vi "MiPS_switch_heater.vi"(0 "ref_big_msg":refnum<vi>, 1 "ref_shim_relay_ch1":refnum<vi>, 2 "ref_shim_relay_ch2":refnum<vi>, 4 "ref_shim_relay_status":refnum<vi>, 5 "error in":errorcluster, 6 "ref_timeout_slider":refnum<vi>, 7 "heater_status_now":bool, 8 "ref_in":T1, 9 "ISOBUS address":T4, 10 "switching_allowed":bool, 11 "conn_id_in":refnum<k5>) -> (13 "conn_id_out":refnum<k5>, 14 "ref_out":T1, 19 "error out":errorcluster)   [LabVIEW 2019]
uses:
  Mercury iXX Modules/Public/Controls/ISOBus Address.ctl
  Mercury iXX Modules/Public/Controls/Mercury Reference.ctl
  Mercury iXX Modules/Public/Controls/Comms Transport Layer.ctl
  Mercury iXX Modules/Private/Controls/Query Dynamic Reference.ctl
  Mercury iXX Modules/Public/Libraries/Magnet/Controls/Switch Heater.ctl
  Mercury iXX Modules/Public/Libraries/Magnet/Signals/Set/Switch Heater No Check (Set).vi
  Mercury iXX Modules/Public/Libraries/Magnet.lvlib
  Mercury iXX Modules/Mercury iXX.lvlib
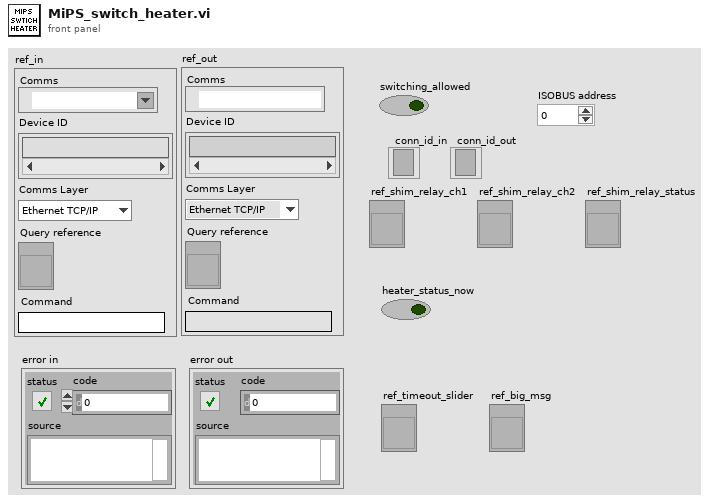
[diagram p1: front panel]
types:
  T1 = typedef "Mercury iXX.lvlib/Mercury Reference.ctl" = cluster{"Comms":refnum<visa-resource-name>, "Device ID":string[], "Comms Layer":T2, "Command":string, "Query reference":T3}
  T2 = typedef "Mercury iXX.lvlib/Comms Transport Layer.ctl" = enum16{"Ethernet TCP/IP", "USB", "ISOBus - RS-232", "GPIB"}
  T3 = typedef "Mercury iXX.lvlib/Query Dynamic Reference.ctl" = refnum<vi>
  T4 = typedef "Mercury iXX.lvlib/ISOBus Address.ctl" = i32
  T5 = typedef "Mercury iXX.lvlib/Magnet.lvlib/Switch Heater.ctl" = string
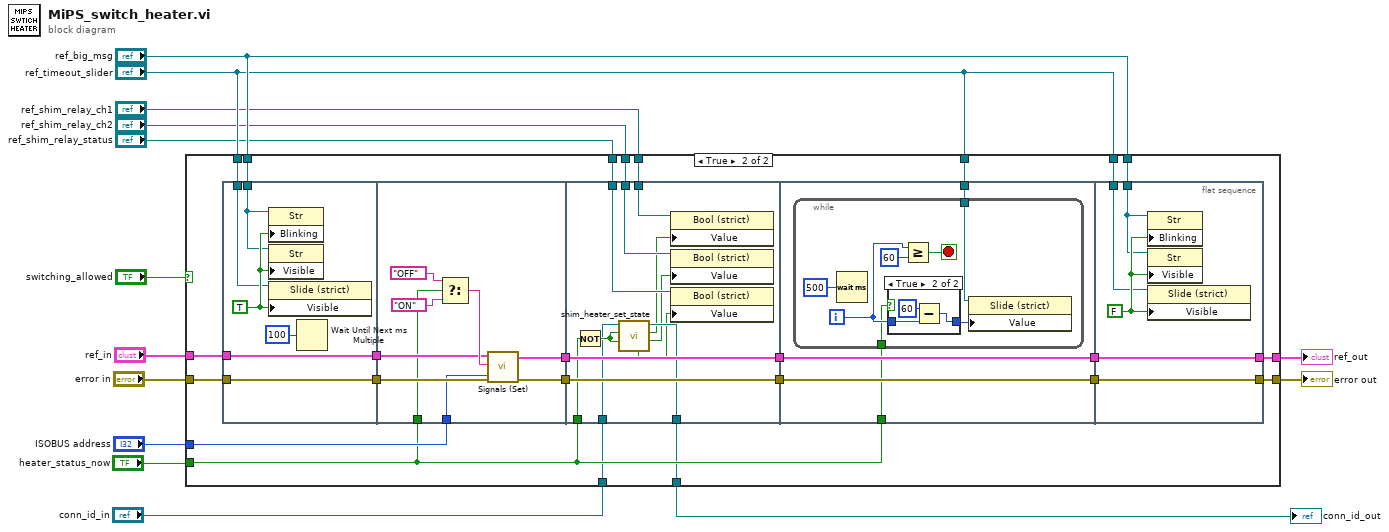
[diagram p0: block diagram]
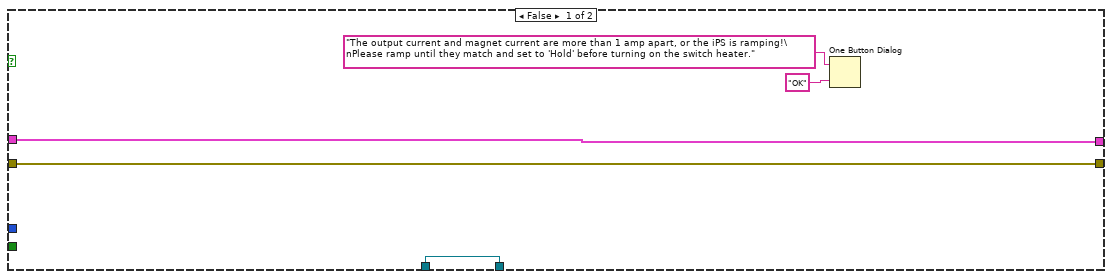
[diagram p2: hidden frame]
diagram:
  n1 = case shown="True" "switching_allowed" {
    tunnel: "heater_status_now" -> [_ w22]
    tunnel: "ref_in" -> [w19 w38]
    tunnel: [w19 w41] -> w10
    tunnel: "error in" -> [w18 w40]
    tunnel: [w18 w39] -> w12
    tunnel: "ISOBUS address" -> [_ w37]
    tunnel: "ref_timeout_slider" -> [_ w30]
    tunnel: "ref_timeout_slider" -> [_ w29]
    tunnel: "ref_big_msg" -> [_ w28]
    tunnel: "ref_big_msg" -> [_ w23]
    tunnel: "ref_timeout_slider" -> [_ w27]
    tunnel: "ref_shim_relay_ch1" -> [_ w26]
    tunnel: "ref_shim_relay_ch2" -> [_ w25]
    tunnel: "ref_shim_relay_status" -> [_ w24]
    tunnel: "conn_id_in" -> [w15 w21]
    tunnel: [w15 w20] -> w1
    frame False {
      n2 = One Button Dialog(message="The output current and magnet current are more than 1 amp apart, or the iPS is ramping!\nPlease ramp until they match and set to 'Hold' before turning on the switch heater.", button name ("OK")="OK") -> ()  [unwired: 1 out]
    }
    frame True {
      n3 = flat-sequence {
        tunnel: [w49] -> w43
        tunnel: w38 -> [w49]
        tunnel: [w47] -> w42
        tunnel: w40 -> [w47]
        tunnel: w28 -> [w45]
        tunnel: w30 -> [w44]
        tunnel: w43 -> [w55]
        tunnel: w42 -> [w53]
        tunnel: [w54] -> w34
        tunnel: [w52] -> w32
        tunnel: w37 -> [w51]
        tunnel: w22 -> [w50]
        tunnel: w34 -> [w70]
        tunnel: [w70] -> w33
        tunnel: w32 -> [w69]
        tunnel: [w69] -> w31
        tunnel: w26 -> [w68]
        tunnel: w25 -> [w67]
        tunnel: w24 -> [w66]
        tunnel: w22 -> [w65]
        tunnel: w21 -> [w63]
        tunnel: [w62] -> w20
        tunnel: w33 -> [w74]
        tunnel: w31 -> [w73]
        tunnel: [w74] -> w36
        tunnel: [w73] -> w35
        tunnel: w29 -> [w72]
        tunnel: w22 -> [w71]
        tunnel: [w89] -> w39
        tunnel: [w90] -> w41
        tunnel: w36 -> [w90]
        tunnel: w35 -> [w89]
        tunnel: w23 -> [w87]
        tunnel: w27 -> [w86]
        frame #0 {
          w46 = TRUE ("Visible")
          n4 = property on="Property Node" class="Str"(reference=w45, "Blinking"=w46) -> ()  [unwired: 1 in, 2 out]
          n5 = property on="Property Node" class="Str"(reference=w45, "Visible"=w46) -> ()  [unwired: 1 in, 2 out]
          n6 = property on="Property Node" class="Slide (strict)"(reference=w44, "Visible"=w46) -> ()  [unwired: 1 in, 2 out]
          n7 = Wait Until Next ms Multiple(millisecond multiple=u32 100) -> ()  [unwired: 1 out]
        }
        frame #1 {
          n8 = Select(t=T5 "OFF" ("Set Switch Heater"), s=w50, f=T5 "ON" ("Set Switch Heater")) -> (s? t:f=w56:T5)
          n9 = call-poly "Signals (Set).vi"("ISOBUS address"=w51, "error in"=w53, "Set Switch Heater"=w56, "Mercury Reference In"=w55) -> ("error out"=w52:errorcluster, "Mercury Reference Out"=w54:T1)  [unwired: 4 in, 2 out]
        }
        frame #2 {
          n10 = Not(x=w65) -> (.not. x?=w64:bool)
          n11 = call "shim_heater_set_state.vi"("state_ch2"=w64, "state_ch1"=w64, "conn_id_in"=w63) -> ("ch2"=w60:bool, "ch1"=w61:bool, "conn_id_out"=w62:refnum<k5>, "status"=w59:bool)  [unwired: 3 in, 2 out]
          n12 = property on="Property Node" class="Bool (strict)"(reference=w68, "Value"=w61) -> ()  [unwired: 1 in, 2 out]
          n13 = property on="Property Node" class="Bool (strict)"(reference=w67, "Value"=w60) -> ()  [unwired: 1 in, 2 out]
          n14 = property class="Bool (strict)"(reference=w66, "Value"=w59) -> ()  [unwired: 1 in, 2 out]
        }
        frame #3 {
          n15 = while {
            tunnel: w72 -> [w76]
            tunnel: w71 -> [w75]
            i -> [w78]
            stop <- w80 stop-if-true
            n16 = Wait (ms)(milliseconds to wait=u32 500) -> ()  [unwired: 1 out]
            n17 = case shown="True" w75 {
              tunnel: [w82 w83] -> w77
              tunnel: w78 -> [w82 w85]
              frame False {
              }
              frame True {
                n18 = Subtract(x=60, y=w85) -> (x-y=w83:i32)
              }
            }
            n19 = Greater Or Equal?(x=w78, y=60) -> (x >= y?=w80:bool)
            n20 = property on="Property Node" class="Slide (strict)"(reference=w76, "Value"=w77) -> ()  [unwired: 1 in, 2 out]
          }
        }
        frame #4 {
          w88 = FALSE ("Visible")
          n21 = property on="Property Node" class="Str"(reference=w87, "Blinking"=w88) -> ()  [unwired: 1 in, 2 out]
          n22 = property on="Property Node" class="Str"(reference=w87, "Visible"=w88) -> ()  [unwired: 1 in, 2 out]
          n23 = property on="Property Node" class="Slide (strict)"(reference=w86, "Visible"=w88) -> ()  [unwired: 1 in, 2 out]
        }
      }
    }
  }
  "error out" <- w12
  "ref_out" <- w10
  "conn_id_out" <- w1
